vi "DrawPoint.vi"(2 "Start":T1=[[1.0, 0.0, 0.0, 0.0], [0.0, 1.0, 0.0, 0.0], [0.0, 0.0, 1.0, 0.0], [0.0, 0.0, 0.0, 1.0]], 3 "Stage in":refnum<vi>) -> (1 "Stage out":refnum<vi>)   [LabVIEW 2018]
uses:
  <vilib>/Analysis/Matrix/Datatypes/RealMatrix.ctl
  <vilib>/picture/3D Picture Control/NI_3D Picture Control.lvlib
  <vilib>/Analysis/Matrix/NI_Matrix.lvlib
panel:
  out "error out":errorcluster
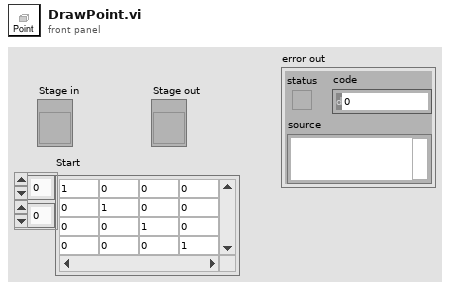
[diagram p1: front panel]
types:
  T1 = typedef "NI_Matrix.lvlib/RealMatrix.ctl" = dbl[][]
  T2 = cluster{"X":sgl, "Y":sgl, "Z":sgl, "Color Box":u32, "Alpha":sgl}
  T3 = cluster{"Start[0]":dbl, "Start[1]":dbl, "Start[2]":dbl}
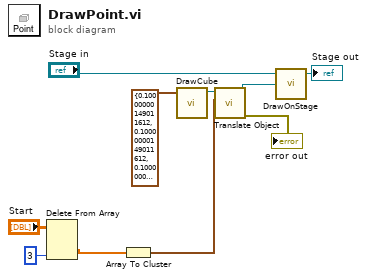
[diagram p0: block diagram]
diagram:
  n1 = Delete From Array(array="Start", index (col)=3 ("disabled index (col)")) -> (deleted portion=w2:dbl[])  [unwired: 2 in, 1 out]
  n2 = Array To Cluster(array=w2) -> (cluster=w4:T3)
  n3 = call "DrawCube.vi"("Cube"=T2 {"X"=0.1, "Y"=0.1, "Z"=0.1, "Color Box"=13816530, "Alpha"=1.0}) -> ("object out"=w7:refnum<vi>)  [unwired: 5 in, 1 out]
  n4 = call <vilib>:"Translate Object.vi"("Translation"=w4, "Scene.Object In"=w7) -> ("error out"=→"error out":errorcluster, "Scene.Object Out"=w6:refnum<vi>)  [unwired: 8 in]
  n5 = call "DrawOnStage.vi"("object in"=w6, "Stage in"="Stage in") -> ("Stage out"=→"Stage out":refnum<vi>)  [unwired: 1 in, 2 out]
